vi "Assign Cluster Element Value by Name.vi"(5 "Element Name":string, 7 "Value":variant, 8 "error in":errorcluster, 11 "Generic Optimization":refnum<class "Generic Optimization.lvclass">) -> (0 "error out":errorcluster, 3 "Generic Optimization out":refnum<class "Generic Optimization.lvclass">)   [LabVIEW 2018, in "Generic Optimization Actor.lvlib" / "Generic Optimization.lvclass"]
uses:
  Generic Optimization.lvclass
  Controls/Optimization Data Cluster.ctl
  Generic Optimization.lvclass/Generic Optimization.ctl
  <vilib>/Utility/Data Type/NI_Data Type.lvlib
panel:
  in  "Optimization Data":T1
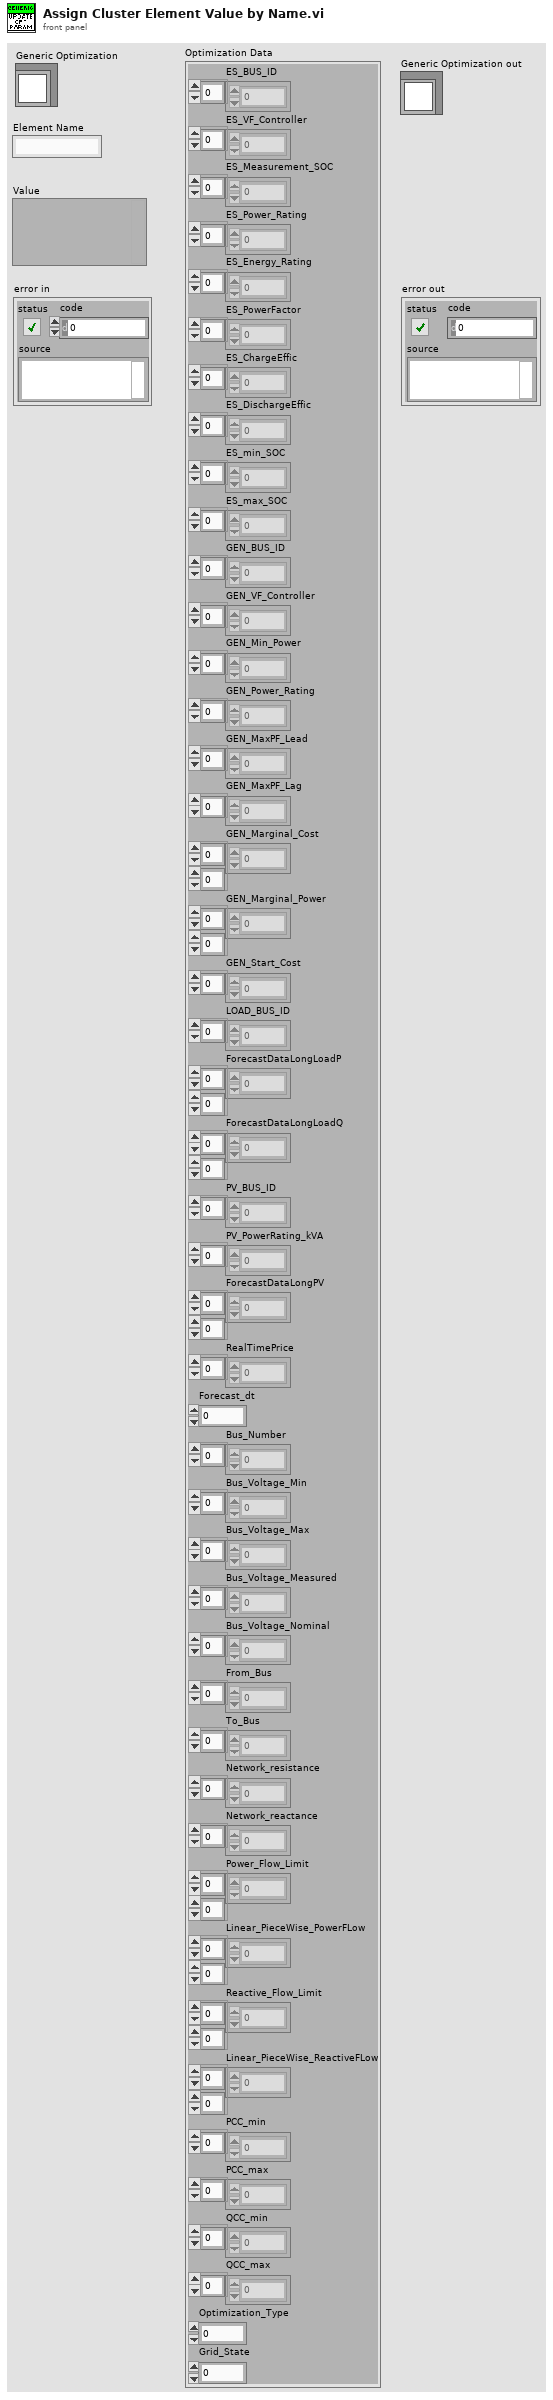
[diagram p1: front panel]
types:
  T1 = typedef "Generic Optimization Actor.lvlib/Generic Optimization.lvclass/Optimization Data Cluster.ctl" = cluster{"ES_BUS_ID":dbl[], "ES_VF_Controller":dbl[], "ES_Measurement_SOC":dbl[], "ES_Power_Rating":dbl[], "ES_Energy_Rating":dbl[], "ES_PowerFactor":dbl[], "ES_ChargeEffic":dbl[], "ES_DischargeEffic":dbl[], "ES_min_SOC":dbl[], "ES_max_SOC":dbl[], "GEN_BUS_ID":dbl[], "GEN_VF_Controller":dbl[], "GEN_Min_Power":dbl[], "GEN_Power_Rating":dbl[], "GEN_MaxPF_Lead":dbl[], "GEN_MaxPF_Lag":dbl[], "GEN_Marginal_Cost":dbl[][], "GEN_Marginal_Power":dbl[][], "GEN_Start_Cost":dbl[], "LOAD_BUS_ID":dbl[], "ForecastDataLongLoadP":dbl[][], "ForecastDataLongLoadQ":dbl[][], "PV_BUS_ID":dbl[], "PV_PowerRating_kVA":dbl[], "ForecastDataLongPV":dbl[][], "RealTimePrice":dbl[], "Forecast_dt":dbl, "Bus_Number":dbl[], "Bus_Voltage_Min":dbl[], "Bus_Voltage_Max":dbl[], "Bus_Voltage_Measured":dbl[], "Bus_Voltage_Nominal":dbl[], "From_Bus":dbl[], "To_Bus":dbl[], "Network_resistance":dbl[], "Network_reactance":dbl[], "Power_Flow_Limit":dbl[][], "Linear_PieceWise_PowerFLow":dbl[][], "Reactive_Flow_Limit":dbl[][], "Linear_PieceWise_ReactiveFLow":dbl[][], "PCC_min":dbl[], "PCC_max":dbl[], "QCC_min":dbl[], "QCC_max":dbl[], "Optimization_Type":i32, "Grid_State":i32}
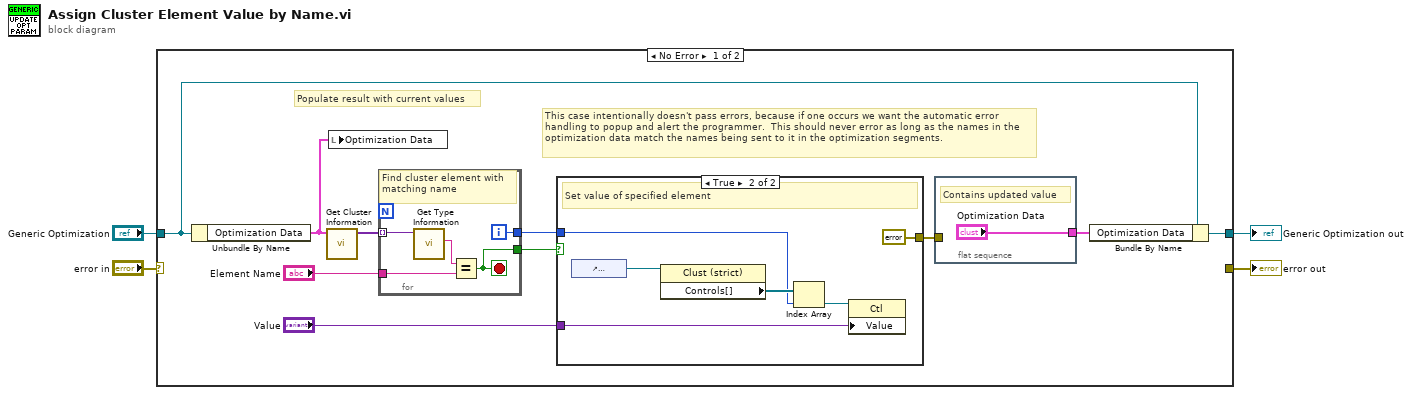
[diagram p0: block diagram]
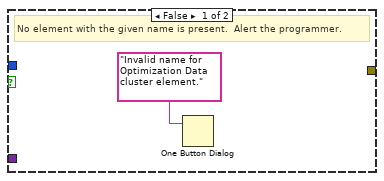
[diagram p2: hidden frame]
diagram:
  n1 = case shown="No Error" "error in" {
    selector: "error in" -> [_ w29]
    tunnel: "Generic Optimization" -> [w7 w28]
    tunnel: [w5 w28] -> w3
    tunnel: [_ w29] -> w1
    frame No Error {
      # "This case intentionally doesn't pass errors, because if one occurs we want the automatic error handling to popup and alert the programmer.  This should never error as long as the names in the optimization data match the names being sent to it in the optimization segments."
      # "Populate result with current values"
      n2 = Unbundle By Name(w7) -> ("Optimization Data"=w8:T1)
      n3 = call <vilib>:"Get Cluster Information.vi"("Variant"=w8) -> ("Cluster Elements"=w14:variant[])  [unwired: 9 in, 1 out]
      n4 = local write "Optimization Data"(w8) -> ()
      n5 = for {
        tunnel: w14 -> [w27] mode=indexing
        tunnel: "Element Name" -> [w26]
        tunnel: [w25] -> w12
        tunnel: [w24] -> w11
        i -> [w25]
        stop <- w24 stop-if-true
        # "Find cluster element with matching name"
        n6 = call <vilib>:"Get Type Information.vi"("Variant"=w27) -> ("Name"=w23:string)  [unwired: 6 in, 4 out]
        n7 = Equal?(x=w23, y=w26) -> (x = y?=w24:bool)
      }
      n8 = case shown="True" w11 {
        tunnel: w12 -> [_ w21]
        tunnel: "Value" -> [_ w19]
        tunnel: [_ errorcluster {"status"=FALSE, "code"=0, "source"=""} ("error in (no error)")] -> w9
        frame False {
          # "No element with the given name is present.  Alert the programmer."
          n9 = One Button Dialog(message="Invalid name for Optimization Data cluster element.") -> ()  [unwired: 1 in, 1 out]
        }
        frame True {
          # "Set value of specified element"
          n10 = control-ref of="Optimization Data"() -> (w18:refnum<vi>)
          n11 = property class="Clust (strict)"(reference=w18) -> ("Controls[]"=w22:refnum<vi>[])  [unwired: 1 in, 2 out]
          n12 = Index Array(array=w22, index=w21) -> (element=w20:refnum<vi>)
          n13 = property class="Ctl"(reference=w20, "Value"=w19) -> ()  [unwired: 1 in, 2 out]
        }
      }
      n14 = flat-sequence {
        tunnel: w9 -> [_]
        tunnel: ["Optimization Data"] -> w6
        frame #0 {
          # "Contains updated value"
        }
      }
      n15 = Bundle By Name(cluster=w7, "Optimization Data"=w6) -> (w5:refnum<class "Generic Optimization.lvclass">)
    }
    frame Error {
    }
  }
  "Generic Optimization out" <- w3
  "error out" <- w1
